vi "Generate File Name.vi"(5 "slice":i32, 7 "tile":i32) -> (4 "appended path":path, 6 "ret path":path)   [LabVIEW 2018]
uses:
  General/Controls/FGV Actions.ctl
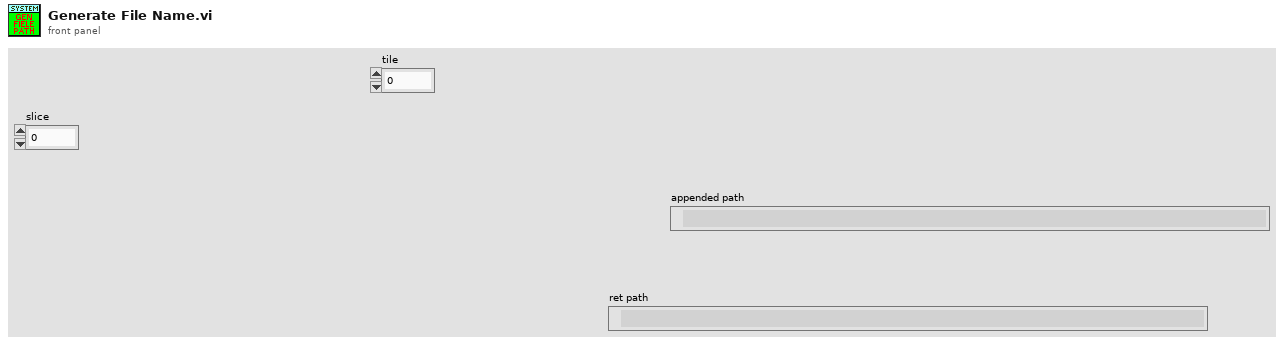
[diagram p1: front panel]
types:
  T1 = enum16{"File name", "X stage", "Y stage", "Slice plane", "Image plane", "time", "output"}
  T2 = typedef "FGV Actions.ctl" = enum16{"Init", "Set", "Get", "Clear"}
  T3 = typedef "System Parameters.ctl" = cluster{"Optical Parameters":T4, "Vibratome":T5, "Table Stages":T6, "Imaging Parameter":T9, "Galvo HW Parameters":cluster{"Analog Out Channel":tag, "Min Voltage":dbl, "Max Voltage":dbl, "Pixel Clock Source":tag, "Sample Rate":dbl, "Line Clock Out Ch":tag}, "Alazar parameters":T11, "Mosaic Paramter":cluster{"X Axis":cluster{"Start [mm]":dbl, "Steps [pts]":dbl, "End [mm]":dbl}, "Y Axis":cluster{"Start [mm]":dbl, "Steps [pts]":dbl, "End [mm]":dbl}, "Scan Pattern":enum16{"Uni-directional", "Bi-Directional", "Spiral Out", "Spiral In"}, "Overlap Options":cluster{"Overlap Type":enum16{"No Overlap", "X Only", "Y Only", "X and Y"}, "Percent Overlap":u8, "Justify":enum16{"Start", "Center", "End"}}}, "Manual Controls":T18, "Vibratome Axis":T21}
  T4 = typedef "Optical Parameters.ctl" = cluster{"Obj. Focal Length [mm]":dbl, "Scan Lens EFL[mm]":dbl, "Tube Lens EFL[mm]":dbl, "Galvo V Range (+/-)":dbl, "Galvo Max Half Angle [Deg]":dbl, "Max Galvo Range[%]":dbl}
  T5 = typedef "Vibratome Parameters.ctl" = cluster{"Z Bottom [mm]":dbl, "Pre Cut Dwell [s]":dbl, "Blade Frequency [RPM]":u16, "Slice Speed [mm/s]":dbl, "Post Cut Dwell [s]":dbl, "Ramp Time [s]":dbl, "Start X [mm]":dbl, "Start Y [mm]":dbl, "Slice Length [mm]":dbl, "Slice Axis":enum16{"X Axis", "Y Axis", "Z Axis"}, "Controller VISA Ref":refnum<visa-resource-name>, "Blade Frequency [Hz]":u16, "Analog Out Channel":tag, "Pixel Clock Source":tag}
  T6 = typedef "Translation Stage Parameters.ctl" = cluster{"X Stage":T7, "Y Stage":T7, "Z Stage":T7}
  T7 = typedef "Translation Stage Cluster.ctl" = cluster{"Position":dbl, "Is.Enabled?":bool, "Is.Connected?":bool, "Device SN":string, "AccelerationMaximum":dbl, "VelocityMaximum":dbl, "Acceleration":dbl, "Velocity":dbl, "waitTimeout (ms)":i32, "Model":T8, "Is.Homed?":bool, "MOVE":bool}
  T8 = typedef "Translation Stage Types.ctl" = enum16{"None", "Thorlabs LTS", "Thorlabs MLJ"}
  T9 = typedef "Imaging Parameters.ctl" = cluster{"Raster Scan Direction":T10, "Pixel Dwell Time [Clock Cycles]":u16, "Flyback Time [Clock Cycles]":u16, "XY Center [um]":cluster{"X":dbl, "Y":dbl}, "Pixel Step Size [um] X":dbl, "XY Image Size":enum16{"32 x 32", "64 x 64", "128 x 128", "256 x 256", "512 x 512", "1024 x 1024", "2048 x 2048"}, "Custom":bool, "Custom Size":cluster{"X":u16, "Y":u16}, "Line Averages":u8, "Pixel Step Size [um] Y":dbl}
  T10 = typedef "Scan Direction.ctl" = enum16{"Uni Directional", "Bi Directional", "None"}
  T11 = typedef "Alazar parameters.ctl" = cluster{"Trigger Settings":cluster{"General Trigger Settings":T12, "Trigger Engine 1":T13, "Trigger Engine 2":T13}, "Device ID":T14, "Ch A Input Control":T15, "Ch B Input Control":T15, "Acq Settings":T16, "Capture Clock":T17}
  T12 = typedef "General Trigger Settings.ctl" = cluster{"Trigger Operation":u32, "Coupling ID":u32, "Range ID":u32, "Delay":u32, "Timeout Ticks":u32, "Mode":u32, "Parameter":u32}
  T13 = typedef "Trigger Engine Controls.ctl" = cluster{"Trigger Engine":u32, "Source":u32, "Slope":u32, "Level":u32}
  T14 = typedef "Alazar Device ID.ctl" = cluster{"System ID":u32, "Board ID":u32}
  T15 = typedef "Channel Input Controls.ctl" = cluster{"Channel":u8, "Coupling":u32, "Range":u32, "Impedance":u32}
  T16 = typedef "Alazar Acquisition Settings.ctl" = cluster{"Record Length":u32, "Offset":u32, "Records Per Buffer":u32, "Records Count (Records/Acq)":u32, "Window Type":u32, "Footer":u32, "Samples per record":u32, "Output Format":u32}
  T17 = typedef "Clock Controls.ctl" = cluster{"Sample Rate":u32, "Decimation":u32, "Source":u32, "Edge":u32}
  T18 = typedef "Manual Controls.ctl" = cluster{"Z0":dbl, "First image height":dbl, "Data Path":path, "Save parameters":T19, "Center Galvos":bool, "Acquisition mode":T20, "PSOCT Channel":u32, "Save":bool, "AIP rotation angle":dbl, "ret ds":bool, "Pause?":bool, "Outgoing Mail Server (SMTP)":string, "Email":string, "Password":string, "Carrier 1":enum16{"T-Mobile", "AT&T", "Verizon", "Sprint"}, "phone number 1":string, "Subject":string, "Message":string, "blocker position":enum16{"every two slices", "Nat slices", "None"}, "Carrier 2":enum16{"T-Mobile", "AT&T", "Verizon", "Sprint"}, "phone number 2":string}
  T19 = typedef "FFT parameters.ctl" = cluster{"start pixel":i32, "#pixels to save":i32}
  T20 = typedef "FFT mode.ctl" = enum16{"ThorOCT B line", "ThorOCT Spectral", "ThorOCT FFT", "Alazar B line", "Alazar FFT", "GPU FFT", "Alazar Spectral", "Simulation", "auto adjust focus", "Save all"}
  T21 = typedef "Vibratome Param.ctl" = cluster{"Start [mm](first cut height)":dbl, "slice thickness[um]":dbl, "#slice":u16, "image thickness(um)":dbl, "#images":u16, "30um?":bool}
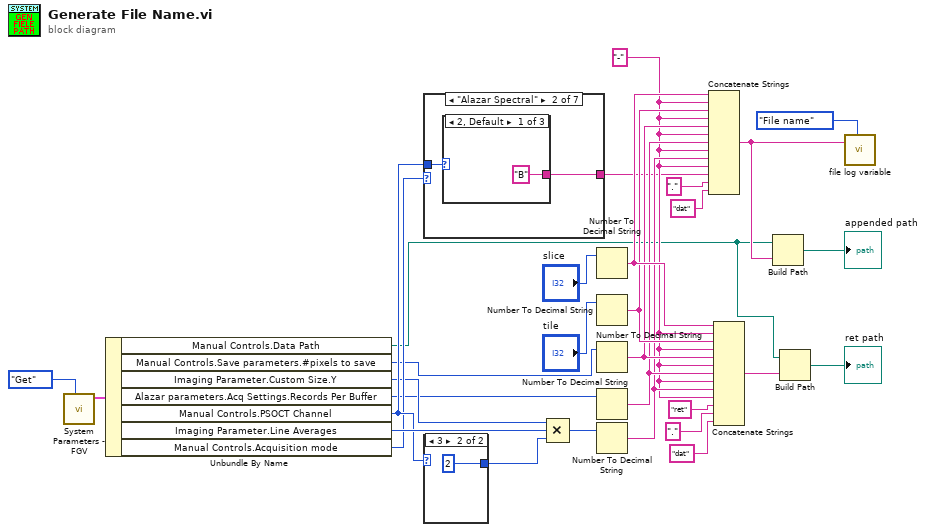
[diagram p0: block diagram]
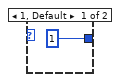
[diagram p2: hidden frame]
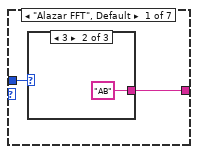
[diagram p3: hidden frame]
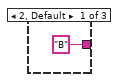
[diagram p4: hidden frame]
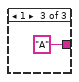
[diagram p5: hidden frame]
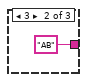
[diagram p6: hidden frame]
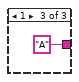
[diagram p7: hidden frame]
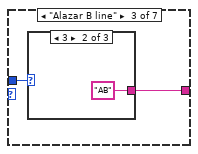
[diagram p8: hidden frame]
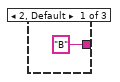
[diagram p9: hidden frame]
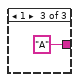
[diagram p10: hidden frame]
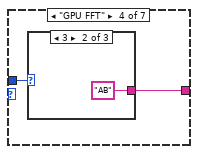
[diagram p11: hidden frame]
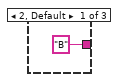
[diagram p12: hidden frame]
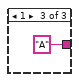
[diagram p13: hidden frame]
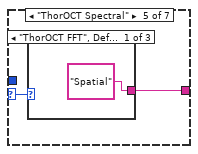
[diagram p14: hidden frame]
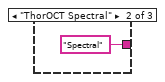
[diagram p15: hidden frame]
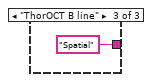
[diagram p16: hidden frame]
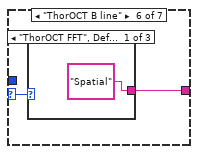
[diagram p17: hidden frame]
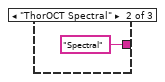
[diagram p18: hidden frame]
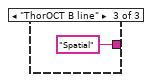
[diagram p19: hidden frame]
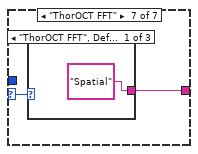
[diagram p20: hidden frame]
diagram:
  w4 = "-" ("string")
  n1 = call "System Parameters - FGV.vi"("Actions"=FGV_Actions."Get") -> ("System Parameters [Out]"=w22:T3)  [unwired: 9 in, 1 out]
  n2 = Unbundle By Name(w22) -> ("Manual Controls.Data Path"=w1:path, "Manual Controls.Save parameters.#pixels to save"=w18:i32, "Imaging Parameter.Custom Size.Y"=w19:u16, "Alazar parameters.Acq Settings.Records Per Buffer"=w17:u32, "Manual Controls.PSOCT Channel"=w21:u32, "Imaging Parameter.Line Averages"=w25:u8, "Manual Controls.Acquisition mode"=w20:T20)
  n3 = case shown="\"Alazar Spectral\"" w20 {
    selector: w20 -> [_ _ _ _ w51 w56 w61]
    tunnel: [w32 w37 w42 w47 w52 w57 w62] -> w3
    tunnel: w21 -> [w31 w36 w41 w46 _ _ _]
    frame "Alazar FFT", Default {
      n4 = case shown="3" w31 {
        tunnel: ["B" "AB" "A"] -> w32
        frame 2, Default {
        }
        frame 3 {
        }
        frame 1 {
        }
      }
    }
    frame "Alazar Spectral" {
      n5 = case shown="2, Default" w36 {
        tunnel: ["B" "AB" "A"] -> w37
        frame 2, Default {
        }
        frame 3 {
        }
        frame 1 {
        }
      }
    }
    frame "Alazar B line" {
      n6 = case shown="3" w41 {
        tunnel: ["B" "AB" "A"] -> w42
        frame 2, Default {
        }
        frame 3 {
        }
        frame 1 {
        }
      }
    }
    frame "GPU FFT" {
      n7 = case shown="3" w46 {
        tunnel: ["B" "AB" "A"] -> w47
        frame 2, Default {
        }
        frame 3 {
        }
        frame 1 {
        }
      }
    }
    frame "ThorOCT Spectral" {
      n8 = case shown="\"ThorOCT FFT\", Default" w51 {
        tunnel: ["Spatial" "Spectral" "Spatial"] -> w52
        frame "ThorOCT FFT", Default {
        }
        frame "ThorOCT Spectral" {
        }
        frame "ThorOCT B line" {
        }
      }
    }
    frame "ThorOCT B line" {
      n9 = case shown="\"ThorOCT FFT\", Default" w56 {
        tunnel: ["Spatial" "Spectral" "Spatial"] -> w57
        frame "ThorOCT FFT", Default {
        }
        frame "ThorOCT Spectral" {
        }
        frame "ThorOCT B line" {
        }
      }
    }
    frame "ThorOCT FFT" {
      n10 = case shown="\"ThorOCT FFT\", Default" w61 {
        tunnel: ["Spatial" "Spectral" "Spatial"] -> w62
        frame "ThorOCT FFT", Default {
        }
        frame "ThorOCT Spectral" {
        }
        frame "ThorOCT B line" {
        }
      }
    }
  }
  n11 = case shown="3" w21 {
    tunnel: [1 2] -> w24
    frame 1, Default {
    }
    frame 3 {
    }
  }
  n12 = Compound Arithmetic op=MULTIPLY(w19, w25, w24) -> (w16:i32)
  n13 = Number To Decimal String(number="slice") -> (decimal integer string=w9:string)  [unwired: 1 in]
  n14 = Number To Decimal String(number="tile") -> (decimal integer string=w8:string)  [unwired: 1 in]
  n15 = Number To Decimal String(number=w18) -> (decimal integer string=w7:string)  [unwired: 1 in]
  n16 = Number To Decimal String(number=w17) -> (decimal integer string=w6:string)  [unwired: 1 in]
  n17 = Number To Decimal String(number=w16) -> (decimal integer string=w5:string)  [unwired: 1 in]
  n18 = Concatenate Strings(w9, w4, w8, w4, w7, w4, w6, w4, w5, w4, w3, "." ("string"), "dat" ("string")) -> (w14:string)
  n19 = Concatenate Strings(w9, w4, w8, w4, w7, w4, w6, w4, w5, w4, "ret" ("string"), "." ("string"), "dat" ("string")) -> (w10:string)
  n20 = Build Path(base path=w1, name or relative path=w14) -> (appended path=→"appended path":path)
  n21 = Build Path(base path=w1, name or relative path=w10) -> (appended path=→"ret path":path)
  n22 = call "file log variable.vi"("file name"=w14, "Item"=T1."File name") -> ()  [unwired: 16 in, 2 out]
